vi "Size0001.vi"   [LabVIEW 2013]
uses:
  <vilib>/Heliosphere Research LLC/Advanced Plotting Toolkit/typedefs/PlotID.ctl
  ErrorCodes.ctl
  <vilib>/Heliosphere Research LLC/Advanced Plotting Toolkit/Advanced Plotting Toolkit.lvlib
types:
  T1 = typedef "ErrorCodes.ctl" = u32
  T2 = typedef "Advanced Plotting Toolkit.lvlib/PlotID.ctl" = i32
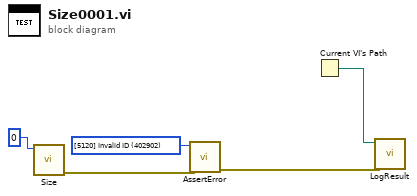
[diagram p0: block diagram]
diagram:
  w1 = T1 402902 items=["[5120] Invalid ID"=402902, "[5110] Failed to Init"=402900, "[5111] Unknown Error"=402901, "[5130] Save - Bad File Extension"=402403, "[5131] Save - General Error"=402904, "[5140] Unsupported (Polar)"=402905, "[5141] Unsupported (Logscale)"=402906, "[5142] Coordinates Not Regular"=402907] ("Expected Error")
  n1 = call <vilib>:"Size.vi"("Plot ID"=T2 0 ("Plot ID In")) -> ("error out"=w2:errorcluster)  [unwired: 9 in, 1 out]
  n2 = call "AssertError.vi"("error in (no error)"=w2, "Expected Error"=w1) -> ("error out"=w4:errorcluster)  [unwired: 9 in]
  n3 = Current VI's Path() -> (path=w5:path)
  n4 = call "LogResult.vi"("Test Result"=w4, "VI Path"=w5) -> ()  [unwired: 10 in]
